vi "wrap.PushChunk.vi"(0 "class.GLue in":refnum<class "class.GLue.lvclass">, 2 "Script":string, 11 "error in (no error)":errorcluster, 13 "Name":string) -> (4 "class.GLue out":refnum<class "class.GLue.lvclass">, 15 "error out":errorcluster)   [LabVIEW 2014, in "GLue.lvlib" / "class.GLue.lvclass"]
uses:
  class.GLue.lvclass
  class.GLue.lvclass/class.GLue.ctl
  Resources/GLue.dll
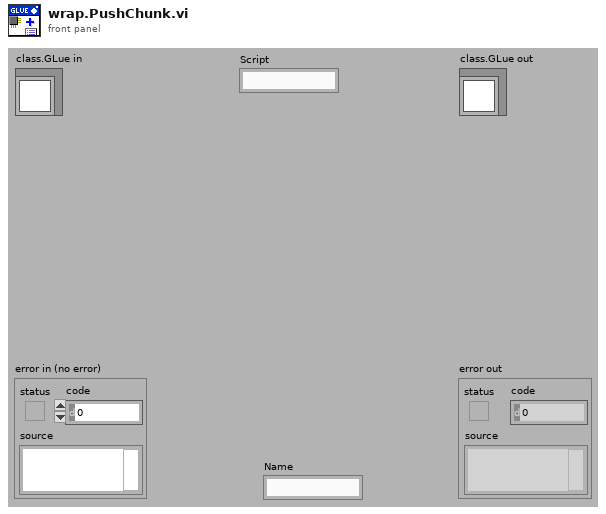
[diagram p1: front panel]
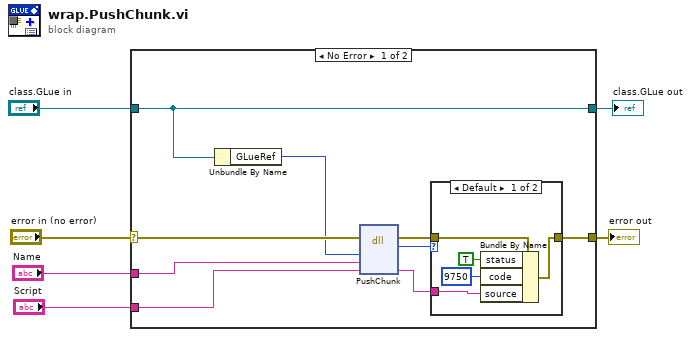
[diagram p0: block diagram]
diagram:
  n1 = case shown="No Error" "error in (no error)" {
    selector: "error in (no error)" -> [w14 w23]
    tunnel: [w8 w23] -> w5
    tunnel: [w15 w22] -> w3
    tunnel: "class.GLue in" -> [w15 w22]
    tunnel: "Name" -> [w12 _]
    tunnel: "Script" -> [w11 _]
    frame No Error {
      n2 = Unbundle By Name(w15) -> ("GLueRef"=w13:i64)
      n3 = dll-call lib="C:/Users/Antonie/Documents/work/glue/trunk/Resources/GLue.dll" fn="PushChunk"(error in=w14, "GLue"=w13, "Name"=w12, "Script"=w11) -> (error out=w9:errorcluster, "return type"=w10:i32, "Script"=w7:string)  [unwired: 4 in, 1 out]
      n4 = case shown="Default" w10 {
        tunnel: w9 -> [w20 w21]
        tunnel: [w19 w21] -> w8
        tunnel: w7 -> [w17 _]
        frame Default {
          n5 = Bundle By Name(cluster=w20, "status"=TRUE, "code"=9750, "source"=w17) -> (w19:errorcluster)
        }
        frame 0 {
        }
      }
    }
    frame Error {
    }
  }
  "error out" <- w5
  "class.GLue out" <- w3
